vi "cut_first_points.vi"(1 "time offset":dbl, 2 "waveform in":waveform(dbl)) -> (0 "output waveform":waveform(dbl))   [LabVIEW 2019]
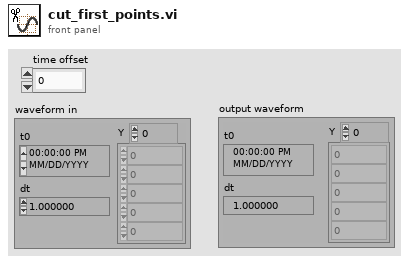
[diagram p1: front panel]
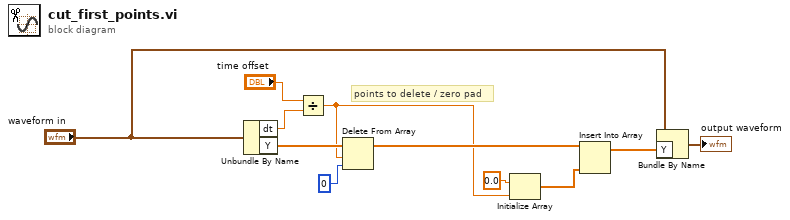
[diagram p0: block diagram]
diagram:
  # "points to delete / zero pad"
  n1 = Unbundle By Name("waveform in") -> ("dt"=w11:dbl, "Y"=w9:dbl[])
  n2 = Divide(x="time offset", y=w11) -> (x/y=w4:dbl)
  n3 = Delete From Array(array=w9, length=w4, index=0) -> (array with subset deleted=w7:dbl[])  [unwired: 1 out]
  n4 = Initialize Array(0.0 ("element"), w4) -> (w6:dbl[])
  n5 = Insert Into Array(array=w7, new element=w6) -> (w3:dbl[])  [unwired: 1 in]
  n6 = Bundle By Name(cluster="waveform in", "Y"=w3) -> (→"output waveform":waveform(dbl))
